vi "Write Connection List.vi"(8 "error in (no error)":errorcluster, 10 "Connection List":string, 11 "Switch Connect Message in":refnum<class "Switch Connect Message.lvclass">) -> (0 "error out":errorcluster, 3 "Switch Connect Message out":refnum<class "Switch Connect Message.lvclass">)   [LabVIEW 2017, in "Messaging.lvlib" / "Switch Connect Message.lvclass"]
uses:
  Switch Connect Message.lvclass
  Switch Connect Message.lvclass/Switch Connect Message.ctl
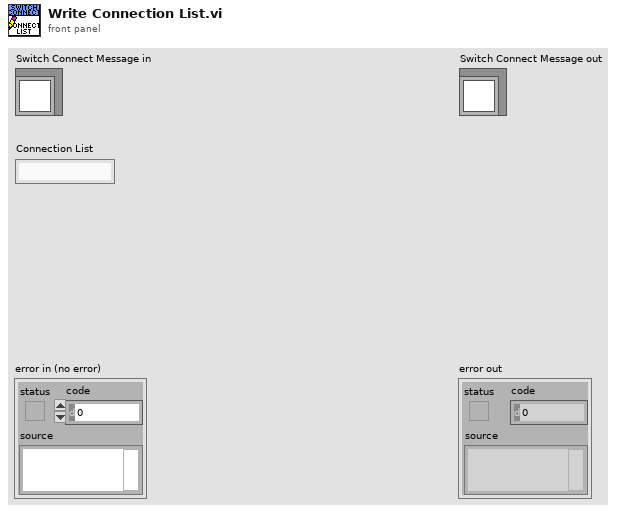
[diagram p1: front panel]
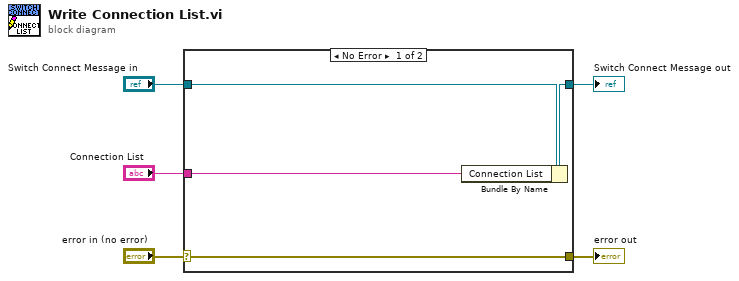
[diagram p0: block diagram]
diagram:
  n1 = case shown="No Error" "error in (no error)" {
    selector: "error in (no error)" -> [w9 w10]
    tunnel: [w9 w10] -> w4
    tunnel: [w7 w11] -> w2
    tunnel: "Switch Connect Message in" -> [w8 w11]
    tunnel: "Connection List" -> [w6 _]
    frame No Error {
      n2 = Bundle By Name(cluster=w8, "Connection List"=w6) -> (w7:refnum<class "Switch Connect Message.lvclass">)
    }
    frame Error {
    }
  }
  "error out" <- w4
  "Switch Connect Message out" <- w2
